vi "RPM probe.vi"() -> ()   [LabVIEW 2016]
uses:
  <vilib>/express/express analysis/Spectral/Block/exnSpectralBlock spectral measurements power poly.vi
  <vilib>/express/express analysis/Spectral/Block/exnSpectralBlock spectral measurements power DDT.vi
  <vilib>/express/express analysis/Spectral/XNode/ExpressSpectralMeasurementsBlockNode.xnode
panel:
  out "Measured Data":dynamicdata(graph)
  out "Power Spectrum":dynamicdata(graph)
  out "Scan number":i32
  in  "Stop":bool
  out "RPM":i32 format="%_5f"
  out "Boolean":bool
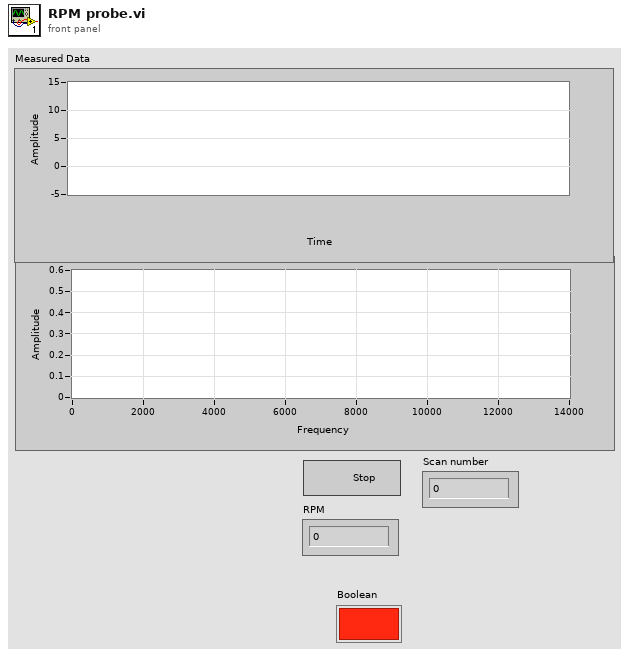
[diagram p1: front panel]
types:
  T1 = cluster{"averaging mode":u16, "weighting mode":u16, "number of averages":u32}
  T2 = cluster{"dB On (F)":bool, "unwrap phase (F)":bool, "convert to degree (F)":bool}
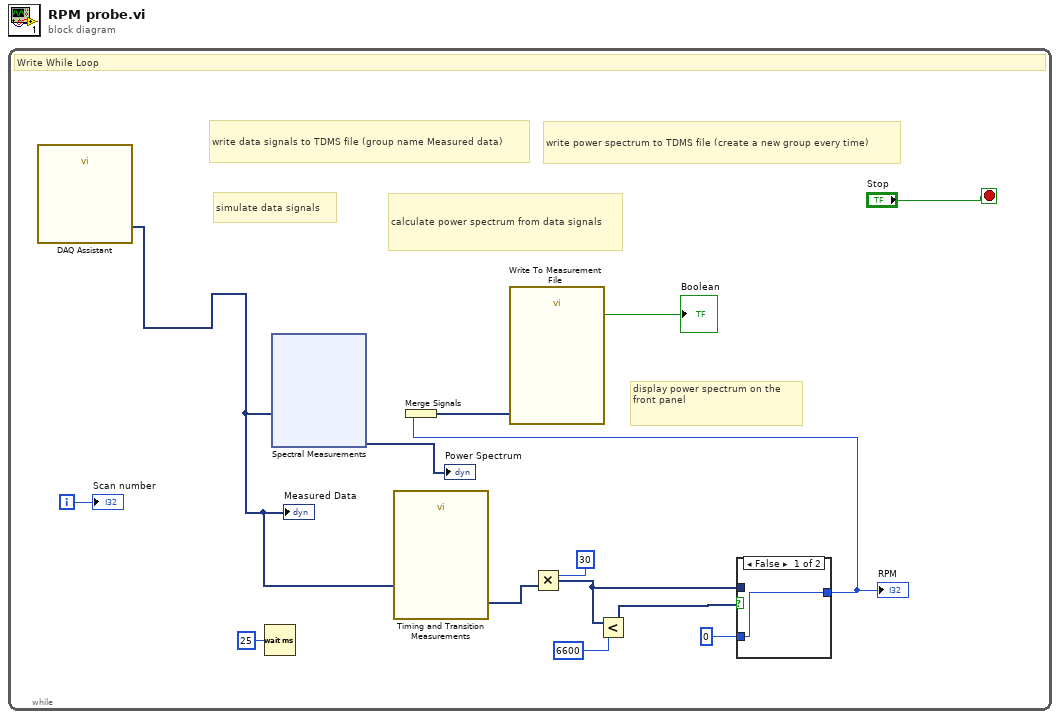
[diagram p0: block diagram]
diagram:
  n1 = while {
    i -> [w14]
    stop <- "Stop" stop-if-true
    # "simulate data signals"
    # "display power spectrum on the front panel"
    # "write power spectrum to TDMS file (create a new group every time)"
    # "calculate power spectrum from data signals"
    # "write data signals to TDMS file (group name Measured data)"
    # "Write While Loop"
    n2 = call "DAQ Assistant"() -> ("data"=w1:dynamicdata)  [unwired: 16 in, 3 out]
    "Measured Data" <- w1
    n3 = Wait (ms)(milliseconds to wait=u32 25) -> ()  [unwired: 1 out]
    n4 = xnode "Spectral Measurements"("Signals"=w1) -> ("Power Spectrum"=→"Power Spectrum":dynamicdata)  [unwired: 1 in, 1 out]
    n5 = call "Timing and Transition Measurements"("Signals"=w1) -> ("Frequency"=w11:dynamicdata)  [unwired: 9 in, 1 out]
    n6 = Multiply(x=u32 30 ("milliseconds to wait"), y=w11) -> (x*y=w3:dynamicdata)
    n7 = Less?(x=w3, y=u32 6600 ("milliseconds to wait")) -> (x < y?=w5:dynamicdata)
    n8 = case shown="False" w5 {
      tunnel: u32 0 ("milliseconds to wait") -> [w15 _]
      tunnel: w3 -> [_ w16]
      tunnel: [w15 w16] -> w2
      frame False {
      }
      frame True {
      }
    }
    "RPM" <- w2
    n9 = Merge Signals(w2) -> (w12:dynamicdata)
    n10 = call "Write To Measurement File"("Signals"=w12) -> ("Saving Data"=→"Boolean":bool)  [unwired: 16 in, 2 out]
    "Scan number" <- w14
  }
